vi "1553B_RECV.vi"(8 "错误输入（无错误）":errorcluster, 10 "IntSource":u32, 11 "VISA资源名称输入":refnum<visa-resource-name>) -> (0 "error out 2":errorcluster, 3 "VISA资源名称输出":refnum<visa-resource-name>)   [LabVIEW 2012]
uses:
  <vilib>/GPower/VIRegister/Library/SubVIs/FindRegisterData.vi
  <vilib>/GPower/VIRegister/Library/SubVIs/WriteSub.vi
  <vilib>/GPower/VIRegister/Library/QManager/GetRegisterData.vi
  <vilib>/GPower/Error/Library/SetError.vi
  <vilib>/GPower/Error/Library/FilterCodes.vi
  <vilib>/GPower/Error/Library/Filter/FilterMulti.vi
  <vilib>/GPower/VIRegister/Library/QManager/QManagerAction.vi
  <vilib>/GPower/Error/Library/ErrorType.vi
  <vilib>/GPower/Error/Library/SplitAppended.vi
  <vilib>/GPower/Error/Library/SubVIs/ExplanationToError.vi
  com/TONGXUN/write32.vi
  <vilib>/GPower/VIRegister/Library/QManager/GetQName.vi
  <vilib>/GPower/VIRegister/Library/QManager/StartQManager.vi
  <vilib>/Utility/error.llb/Trim Whitespace.vi
  <vilib>/dlg_ctls.llb/Space Constant.vi
  <vilib>/Utility/error.llb/Error Code Database.vi
  <vilib>/GPower/Error/Library/SubVIs/SetStatus.vi
  <vilib>/GPower/Error/Library/AppendErrors.vi
  <vilib>/GPower/Error/Library/Append/AppendSingle.vi
  <vilib>/GPower/VIRegister/VIRegister.lvlib
panel:
  out "U8 3":u8[](array[numeric]) format="%.0x"
  out "U8 2":u8[](array[numeric]) format="%.0x"
  out "U8":u8[](array[numeric]) format="%.0x"
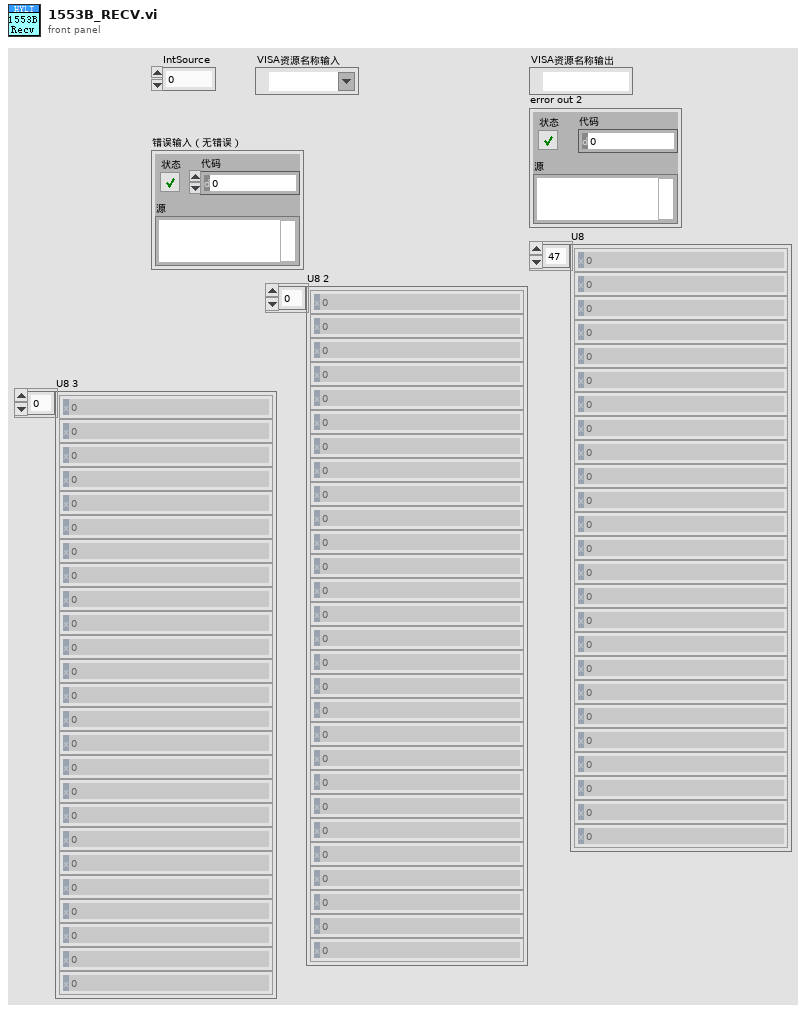
[diagram p1: front panel]
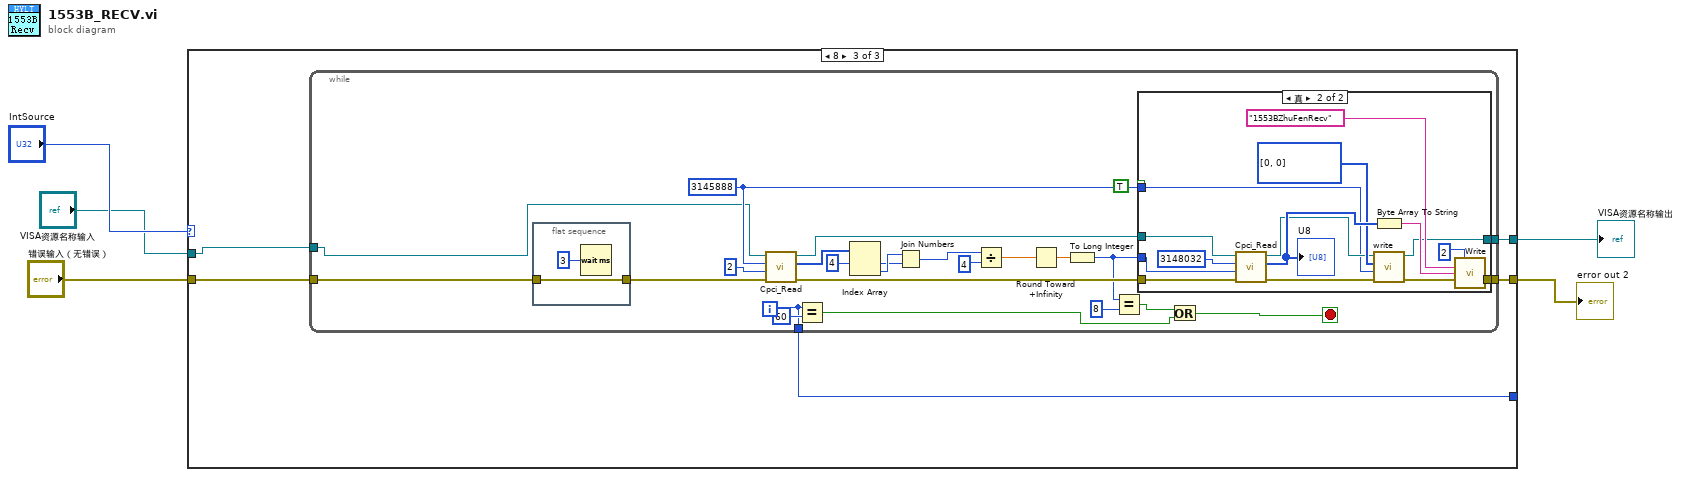
[diagram p0: block diagram]
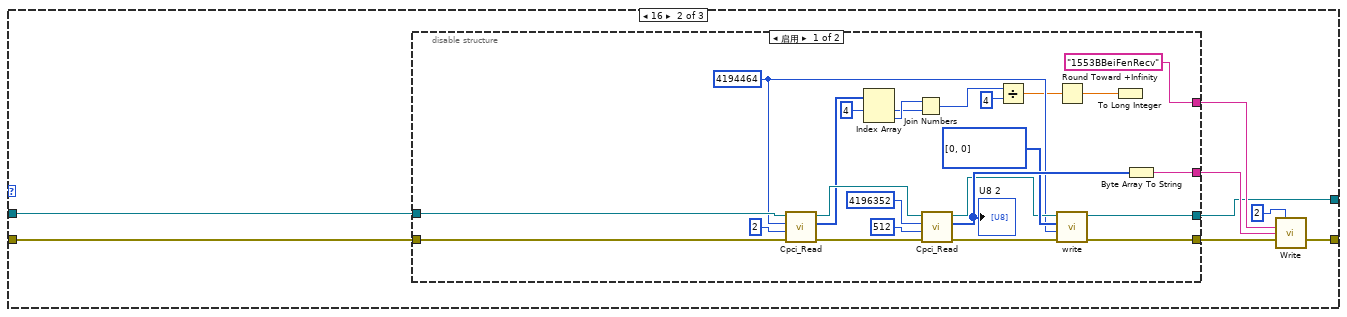
[diagram p3: hidden frame]
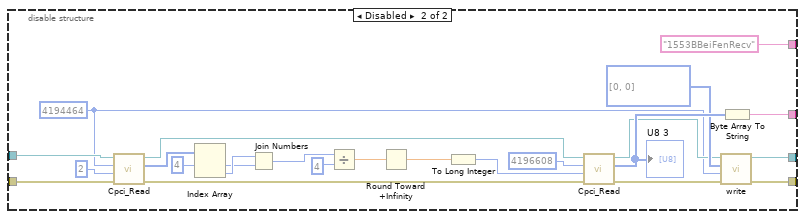
[diagram p4: hidden frame]
diagram:
  n1 = case shown="8" "IntSource" {
    tunnel: "VISA资源名称输入" -> [w7 w13 w64]
    tunnel: [w7 w12 w68] -> w4
    tunnel: "错误输入（无错误）" -> [w6 w11 w65]
    tunnel: [w6 w9 w67] -> w2
    tunnel: [_ _ w66] -> _
    frame 0, Default {
    }
    frame 16 {
      n2 = disable-structure shown="启用" {
        disable-tunnel: ["1553BBeiFenRecv" ("Register name") "1553BBeiFenRecv" ("Register name")] -> w15
        disable-tunnel: [w36 w60] -> w14
        disable-tunnel: w13 -> [w33 w57]
        disable-tunnel: [w21 w44] -> w12
        disable-tunnel: w11 -> [w20 w43]
        disable-tunnel: [w17 w40] -> w10
        frame Enabled {
          w32 = u32 4194464 ("基地址")
          n3 = call "Cpci_Read.vi"("错误输入（无错误）"=w20, "u32_len"=2, "基地址"=w32, "VISA资源名称"=w33) -> ("错误输出"=w19:errorcluster, "U8"=w29:u8[], "VISA资源名称输出"=w30:refnum<visa-resource-name>)  [unwired: 5 in]
          n4 = Index Array(array=w29, index #1=4 ("索引")) -> (element #1=w26:u8, element #2=w27:u8)  [unwired: 1 in]
          n5 = Join Numbers(hi=w27, lo=w26) -> ((hi.lo)=w24:u16)
          n6 = call "Cpci_Read.vi"("错误输入（无错误）"=w19, "u32_len"=512, "基地址"=u32 4196352, "VISA资源名称"=w30) -> ("错误输出"=w18:errorcluster, "U8"=w37:u8[], "VISA资源名称输出"=w34:refnum<visa-resource-name>)  [unwired: 5 in]
          "U8 2" <- w37
          n7 = Divide(x=w24, y=u16 4) -> (x/y=w25:dbl)
          n8 = Round Toward +Infinity(x=w25) -> (ceil(x): smallest int >= x=w22:dbl)
          n9 = call-poly <vilib>:"write.vi"("error out"=w18, "起始地址"=w32, "U32"=u32[] [0, 0], "VISA资源名称输入"=w34) -> ("error out 2"=w17:errorcluster, "VISA资源名称输出"=w21:refnum<visa-resource-name>)  [unwired: 6 in]
          n10 = To Long Integer(number=w22) -> ()  [unwired: 1 out]
          n11 = Byte Array To String(unsigned byte array=w37) -> (string=w36:string)
        }
        frame Disabled {
          w56 = u32 4194464 ("基地址")
          n12 = call "Cpci_Read.vi"("错误输入（无错误）"=w43, "u32_len"=2, "基地址"=w56, "VISA资源名称"=w57) -> ("错误输出"=w42:errorcluster, "U8"=w53:u8[], "VISA资源名称输出"=w54:refnum<visa-resource-name>)  [unwired: 5 in]
          n13 = Index Array(array=w53, index #1=4 ("索引")) -> (element #1=w50:u8, element #2=w51:u8)  [unwired: 1 in]
          n14 = Join Numbers(hi=w51, lo=w50) -> ((hi.lo)=w48:u16)
          n15 = Divide(x=w48, y=u16 4) -> (x/y=w49:dbl)
          n16 = Round Toward +Infinity(x=w49) -> (ceil(x): smallest int >= x=w46:dbl)
          n17 = To Long Integer(number=w46) -> (32bit integer=w45:i32)
          n18 = call "Cpci_Read.vi"("错误输入（无错误）"=w42, "u32_len"=w45, "基地址"=u32 4196608, "VISA资源名称"=w54) -> ("错误输出"=w41:errorcluster, "U8"=w61:u8[], "VISA资源名称输出"=w58:refnum<visa-resource-name>)  [unwired: 5 in]
          "U8 3" <- w61
          n19 = call-poly <vilib>:"write.vi"("error out"=w41, "起始地址"=w56, "U32"=u32[] [0, 0], "VISA资源名称输入"=w58) -> ("error out 2"=w40:errorcluster, "VISA资源名称输出"=w44:refnum<visa-resource-name>)  [unwired: 6 in]
          n20 = Byte Array To String(unsigned byte array=w61) -> (string=w60:string)
        }
      }
      n21 = call <vilib>:"Write.vi"("Timeout"=2, "Register name"=w15, "Register value"=w14, "Error in"=w10) -> ("Error out"=w9:errorcluster)  [unwired: 9 in, 2 out]
    }
    frame 8 {
      n22 = while {
        tunnel: [w82] -> w68
        tunnel: [w80] -> w67
        tunnel: w64 -> [w71]
        tunnel: w65 -> [w70]
        tunnel: [w73] -> w66
        i -> [w73]
        stop <- w74 stop-if-true
        w93 = u32 3145888 ("基地址")
        n23 = flat-sequence {
          tunnel: w70 -> [w112]
          tunnel: [w112] -> w79
          frame #0 {
            n24 = Wait (ms)(milliseconds to wait=u32 3 ("等待时间（毫秒）")) -> ()  [unwired: 1 out]
          }
        }
        n25 = call "Cpci_Read.vi"("错误输入（无错误）"=w79, "u32_len"=2, "基地址"=w93, "VISA资源名称"=w71) -> ("错误输出"=w81:errorcluster, "U8"=w90:u8[], "VISA资源名称输出"=w91:refnum<visa-resource-name>)  [unwired: 5 in]
        n26 = Equal?(x=w73, y=60) -> (x = y?=w75:bool)
        n27 = Index Array(array=w90, index #1=4 ("索引")) -> (element #1=w87:u8, element #2=w88:u8)  [unwired: 1 in]
        n28 = Join Numbers(hi=w88, lo=w87) -> ((hi.lo)=w85:u16)
        n29 = Divide(x=w85, y=u16 4) -> (x/y=w86:dbl)
        n30 = Round Toward +Infinity(x=w86) -> (ceil(x): smallest int >= x=w83:dbl)
        n31 = To Long Integer(number=w83) -> (32bit integer=w78:i32)
        n32 = Equal?(x=w78, y=8) -> (x = y?=w72:bool)
        n33 = case shown="真" TRUE {
          tunnel: w93 -> [_ w104]
          tunnel: w91 -> [w94 w103]
          tunnel: [w94 w102] -> w82
          tunnel: w81 -> [w95 w101]
          tunnel: [w95 w99] -> w80
          tunnel: w78 -> [_ w97]
          frame False {
          }
          frame True {
            n34 = call "Cpci_Read.vi"("错误输入（无错误）"=w101, "u32_len"=w97, "基地址"=u32 3148032, "VISA资源名称"=w103) -> ("错误输出"=w98:errorcluster, "U8"=w108:u8[], "VISA资源名称输出"=w105:refnum<visa-resource-name>)  [unwired: 5 in]
            "U8" <- w108
            n35 = Byte Array To String(unsigned byte array=w108) -> (string=w107:string)
            n36 = call-poly <vilib>:"write.vi"("error out"=w98, "起始地址"=w104, "U32"=u32[] [0, 0], "VISA资源名称输入"=w105) -> ("error out 2"=w100:errorcluster, "VISA资源名称输出"=w102:refnum<visa-resource-name>)  [unwired: 6 in]
            n37 = call <vilib>:"Write.vi"("Timeout"=2, "Register name"="1553BZhuFenRecv", "Register value"=w107, "Error in"=w100) -> ("Error out"=w99:errorcluster)  [unwired: 9 in, 2 out]
          }
        }
        n38 = Or(x=w72, y=w75) -> (x .or. y?=w74:bool)
      }
    }
  }
  "VISA资源名称输出" <- w4
  "error out 2" <- w2
